vi "New Main Log Loop.vi"() -> ()   [LabVIEW 2015]
uses:
  Old code/packet types.ctl
  frc-software-2016/Robot/Main/Robot Global Data.vi
  <vilib>/Rock Robotics/WPI/Solenoid/Deprecated/WPI_SolenoidGetBool.vi
  frc-software-2016/Sprocket/lib/Sprocket.lvlib
  frc-software-2016/Sprocket/src/Refname/Actuators.ctl
panel:
  out "error out":errorcluster
  out "result string":string
  in  "error in (no error)":errorcluster
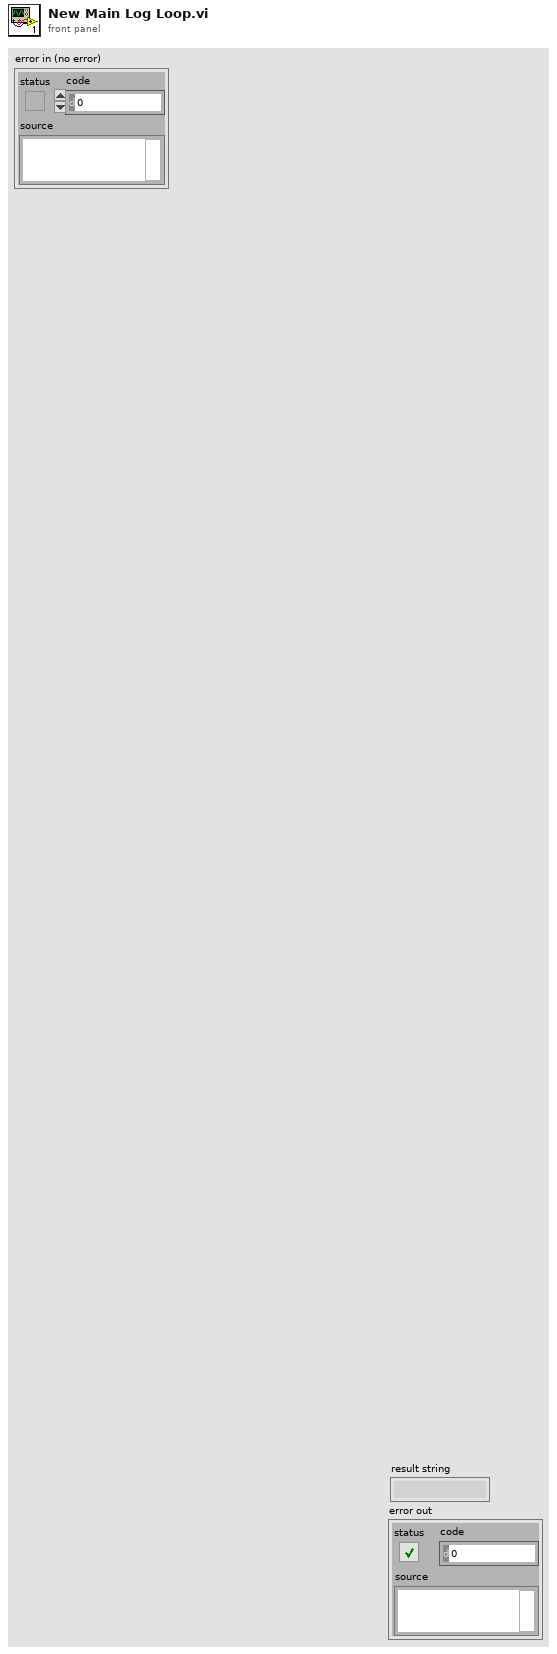
[diagram p1: front panel]
types:
  T1 = typedef "Sprocket.lvlib/Actuators.ctl" = enum16{"Drive Motors L.Top", "Drive Motors R.Top", "Drive Motors L.Bot", "Drive Motors R.Bot", "Collector Motor", "Collector Solenoid", "Compressor", "SonicShifter"}
  T2 = typedef "packet types.ctl" = enum16{"Log line", "Open File", "Send Header", "Set Time", "Send to LCD"}
  T3 = typedef "WPI_SerialPortRef.ctl" = cluster{"DevStatus":errorcluster, "Serial Port Name":refnum<visa-resource-name>}
  T4 = typedef "WPI_MotorControlDeviceRef.ctl" = cluster{"DeviceStatus":errorcluster, "Type":T5, "PWM":cluster{"PWM Channel":T6, "DeadBand":T7}, "CAN":cluster{"Device Number":u8, "Control Mode":T8, "Semaphore":T9, "Max Vout":dbl, "TalonSRX Control Mode":T10}, "Invert":bool}
  T5 = typedef "WPI_MotorControlType.ctl" = enum16{"PWM", "CAN", "CANTalonSRX"}
  T6 = typedef "FPGA_DIOPWMChannel.ctl" = enum8{"PWM 0", "PWM 1", "PWM 2", "PWM 3", "PWM 4", "PWM 5", "PWM 6", "PWM 7", "PWM 8", "PWM 9", "PWM MXP 0", "PWM MXP 1", "PWM MXP 2", "PWM MXP 3", "PWM MXP 4", "PWM MXP 5", "PWM MXP 6", "PWM MXP 7", "PWM MXP 8", "PWM MXP 9", "Invalid"}
  T7 = typedef "WPI_PWMDeadband.ctl" = cluster{"Name":string, "maxPositivePwm":i32, "minPositivePwm":i32, "centerPwm":i32, "maxNegativePwm":i32, "minNegativePwm":i32, "angularRange":u16}
  T8 = typedef "WPI_CANJaguar_ControlMode.ctl" = enum8{"Percent VBus", "Current", "Speed", "Position", "Voltage"}
  T9 = typedef "Semaphore RefNum" = refnum<k1>
  T10 = typedef "WPI_CANTalonSRX_APIControlMode.ctl" = enum8{"Percent VBus", "Speed", "Position", "Slave", "Unchanged / Invalid", "Voltage Compensation", "Current", "Motion Profile"}
  T11 = typedef "WPI_CompressorDevRef.ctl" = cluster{"DevStatus":errorcluster, "Pneumatics Control Module":u8}
  T12 = typedef "WPI_SolenoidDevRef.ctl" = cluster{"DevStatus":errorcluster, "Pneumatics Control Module":u8, "Forward Solenoid Channel":T13, "Reverse Solenoid Channel":T13}
  T13 = typedef "WPI_SolenoidChannel.ctl" = enum8{"Solenoid 0", "Solenoid 1", "Solenoid 2", "Solenoid 3", "Solenoid 4", "Solenoid 5", "Solenoid 6", "Solenoid 7", "Invalid"}
  T14 = typedef "WPI_DriverStationRobotMode2.ctl" = enum16{"Autonomous Disabled", "Autonomous Enabled", "Teleop Disabled", "Teleop Enabled", "Disconnected", "Finish", "Test Disabled", "Test Enabled", "Emergency Stopped"}
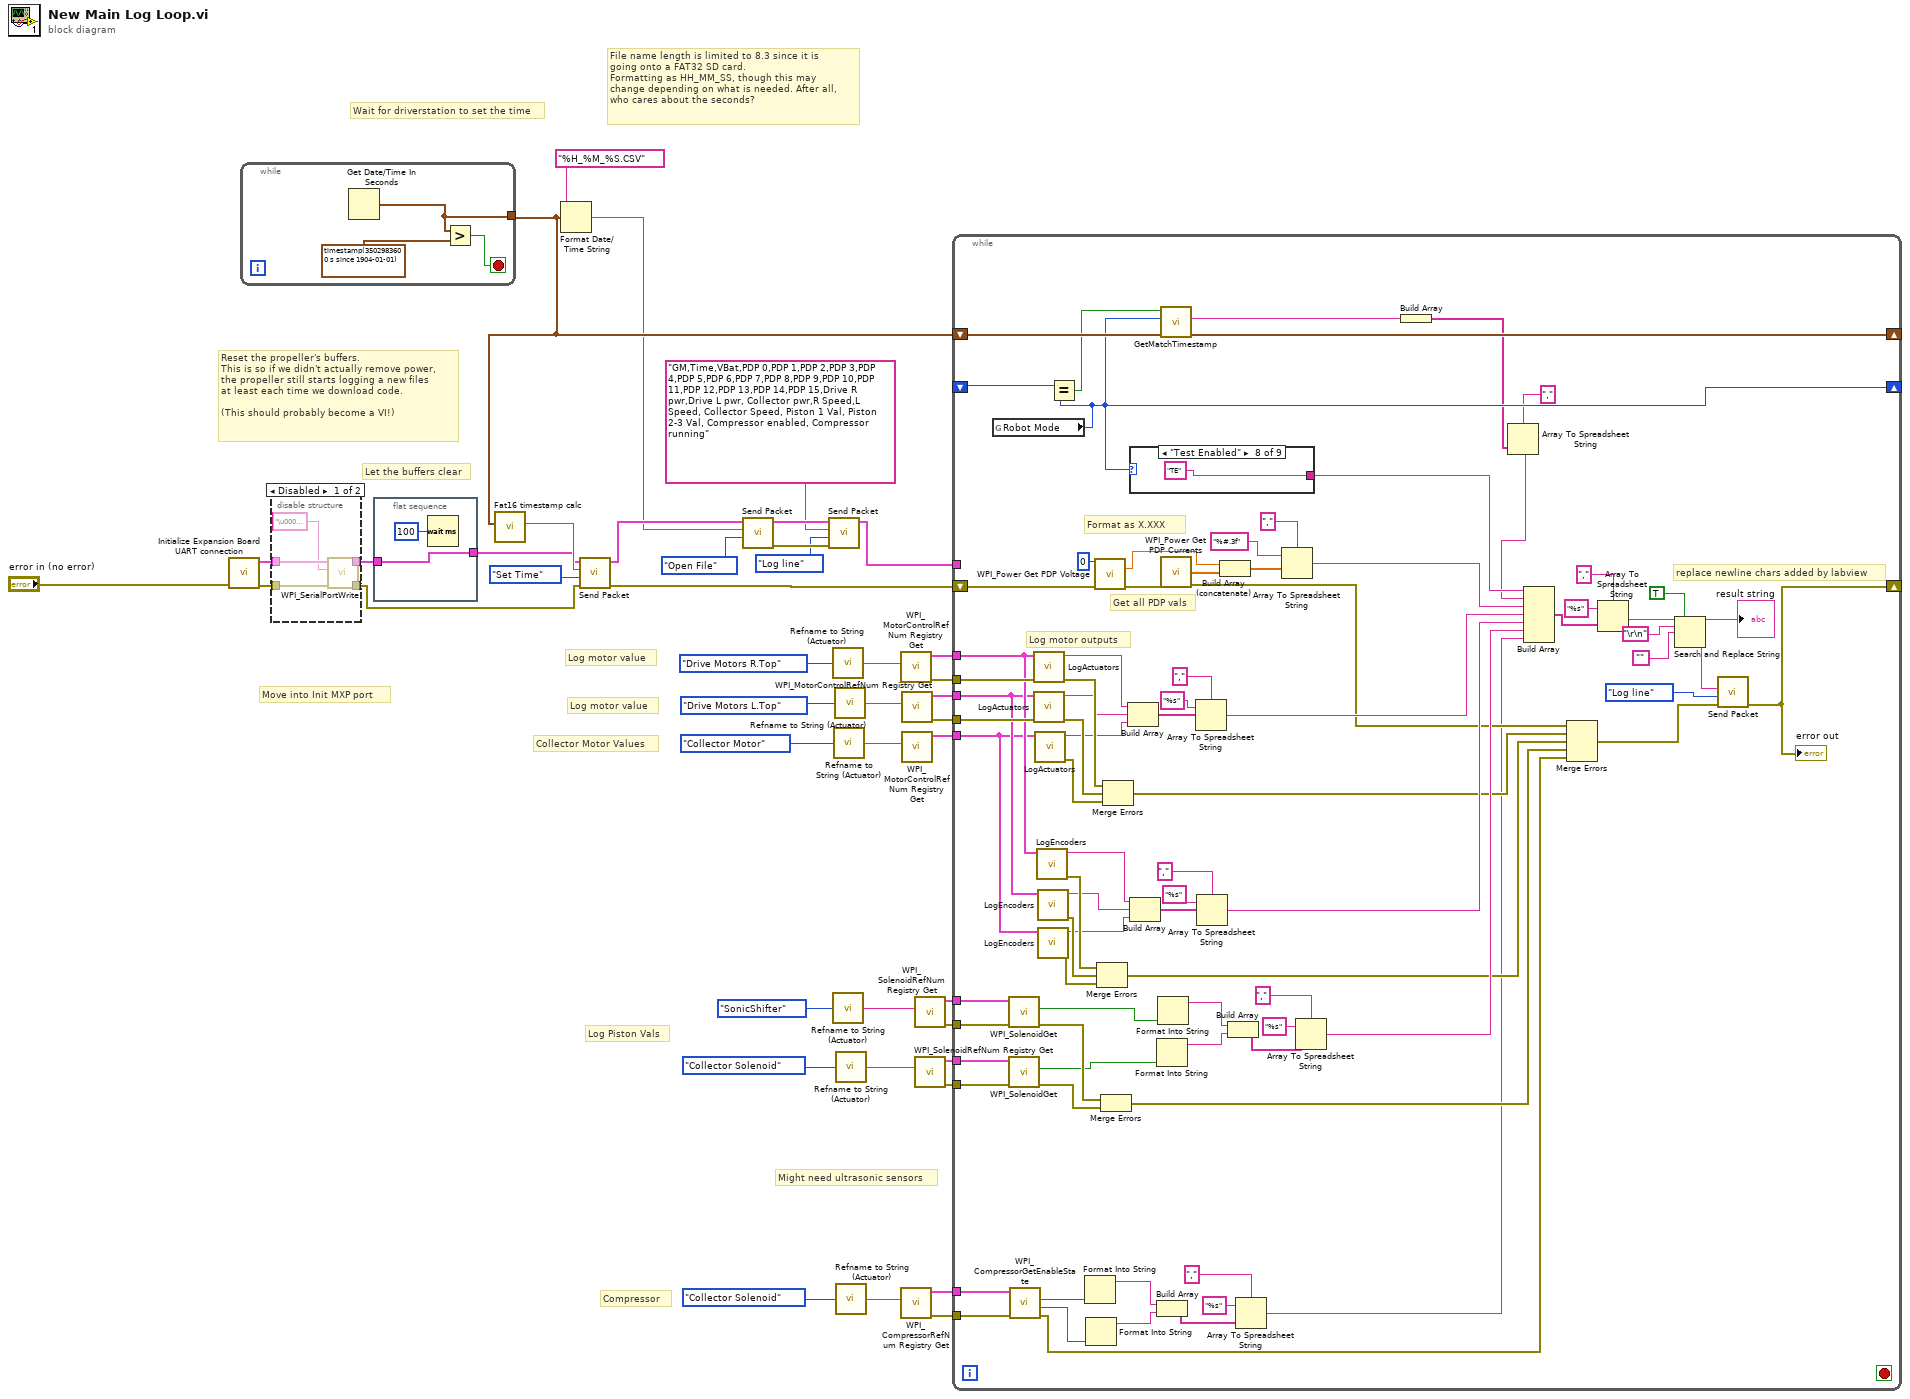
[diagram p0: block diagram]
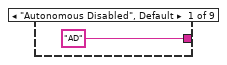
[diagram p2: hidden frame]
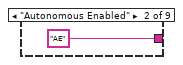
[diagram p3: hidden frame]
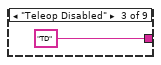
[diagram p4: hidden frame]
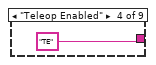
[diagram p5: hidden frame]
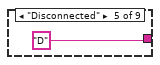
[diagram p6: hidden frame]
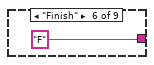
[diagram p7: hidden frame]
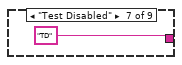
[diagram p8: hidden frame]
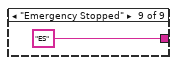
[diagram p9: hidden frame]
diagram:
  # "Might need ultrasonic sensors"
  # "Collector Motor Values"
  # "Compressor"
  # "Log motor value"
  # "Log motor value"
  # "Log Piston Vals"
  # "Move into Init MXP port"
  # "Let the buffers clear"
  # "Reset the propeller's buffers.\nThis is so if we didn't actually remove power,\nthe propeller still starts logging a new files \nat least each time we download code.\n\n(This should probably become a VI!)"
  # "File name length is limited to 8.3 since it is \ngoing onto a FAT32 SD card. \nFormatting as HH_MM_SS, though this may\nchange depending on what is needed. After all,\nwho cares about the seconds?"
  # "Wait for driverstation to set the time"
  n1 = call "Initialize Expansion Board UART connection.vi"("error in (no error)"="error in (no error)") -> ("error out"=w39:errorcluster, "SerialPortRef"=w38:T3)  [unwired: 9 in]
  n2 = while {
    tunnel: [w43] -> w33
    stop <- w44 stop-if-true
    n3 = Get Date/Time In Seconds() -> (seconds since 1Jan1904=w43:timestamp)
    n4 = Greater?(x=w43, y=timestamp(3502983600 s since 1904-01-01)) -> (0:w44:bool)
  }
  n5 = disable-structure shown="Disabled" {
    disable-tunnel: w39 -> [w50 w51]
    disable-tunnel: w38 -> [w49 w52]
    disable-tunnel: [w47 w52] -> w36
    disable-tunnel: [w46 w51] -> w35
    frame Disabled {
      n6 = call <vilib>:"WPI_SerialPortWrite.vi"("error in (no error)"=w50, "Buffer"="\u0004\u0004", "SerialPortRef"=w49) -> ("error out"=w46:errorcluster, "SerialPortRef"=w47:T3)  [unwired: 6 in, 1 out]
    }
    frame Enabled {
    }
  }
  n7 = flat-sequence {
    tunnel: [w54] -> w37
    tunnel: w36 -> [w54]
    frame #0 {
      n8 = Wait (ms)(milliseconds to wait=u32 100) -> ()  [unwired: 1 out]
    }
  }
  n9 = call "Fat16 timestamp calc.vi"("time stamp"=w33) -> ("timestamp as string"=w41:string)  [unwired: 10 in]
  n10 = Format Date/Time String(time format string (%c)="%H_%M_%S.CSV", seconds (now)=w33) -> (date/time string=w26:string)  [unwired: 1 in]
  n11 = call "Send Packet.vi"("error in (no error)"=w35, 7:packet_types."Set Time", "Log string"=w41, "SerialPortRef"=w37) -> ("error out"=w24:errorcluster, "SerialPortRef out"=w27:T3)  [unwired: 4 in]
  n12 = call "Send Packet.vi"(7:packet_types."Open File", "Log string"=w26, "SerialPortRef"=w27) -> ("error out"=w31:errorcluster, "SerialPortRef out"=w32:T3)  [unwired: 5 in]
  n13 = call "Send Packet.vi"("error in (no error)"=w31, 7:packet_types."Log line", "Log string"="GM,Time,VBat,PDP 0,PDP 1,PDP 2,PDP 3,PDP 4,PDP 5,PDP 6,PDP 7,PDP 8,PDP 9,PDP 10,PDP 11,PDP 12,PDP 13,PDP 14,PDP 15,Drive R pwr,Drive L pwr, Collector pwr,R Speed,L Speed, Collector Speed, Piston 1 Val, Piston 2-3 Val, Compressor enabled, Compressor running", "SerialPortRef"=w32) -> ("SerialPortRef out"=w28:T3)  [unwired: 4 in, 1 out]
  n14 = call "Refname to String (Actuator).vi"("Actuator Refname"=Actuators."Drive Motors R.Top") -> ("Refnum Name"=w21:string)
  n15 = call "Refname to String (Actuator).vi"("Actuator Refname"=Actuators."SonicShifter") -> ("Refnum Name"=w11:string)
  n16 = call "Refname to String (Actuator).vi"("Actuator Refname"=Actuators."Collector Motor") -> ("Refnum Name"=w14:string)
  n17 = call "Refname to String (Actuator).vi"("Actuator Refname"=Actuators."Drive Motors L.Top") -> ("Refnum Name"=w19:string)
  n18 = call "Refname to String (Actuator).vi"("Actuator Refname"=Actuators."Collector Solenoid") -> ("Refnum Name"=w7:string)
  n19 = call "Refname to String (Actuator).vi"("Actuator Refname"=Actuators."Collector Solenoid") -> ("Refnum Name"=w2:string)
  n20 = call <vilib>:"WPI_MotorControlRefNum Registry Get.vi"("refnum name"=w21) -> ("error out"=w17:errorcluster, "MotorControlDevRef"=w22:T4)  [unwired: 9 in]
  n21 = call <vilib>:"WPI_CompressorRefNum Registry Get.vi"("refnum name"=w2) -> ("error out"=w1:errorcluster, "CompressorDevRef"=w3:T11)  [unwired: 9 in]
  n22 = call <vilib>:"WPI_MotorControlRefNum Registry Get.vi"("refnum name"=w19) -> ("error out"=w16:errorcluster, "MotorControlDevRef"=w18:T4)  [unwired: 9 in]
  n23 = call <vilib>:"WPI_MotorControlRefNum Registry Get.vi"("refnum name"=w14) -> ("MotorControlDevRef"=w13:T4)  [unwired: 9 in, 1 out]
  n24 = call <vilib>:"WPI_SolenoidRefNum Registry Get.vi"("refnum name"=w11) -> ("error out"=w9:errorcluster, "SolenoidDevRef"=w10:T12)  [unwired: 9 in]
  n25 = call <vilib>:"WPI_SolenoidRefNum Registry Get.vi"("refnum name"=w7) -> ("error out"=w5:errorcluster, "SolenoidDevRef"=w8:T12)  [unwired: 9 in]
  n26 = while {
    shift-right: [w135] -> _
    shift-left: w33 -> [w134]
    shift-right: [w131] -> _
    shift-left: _ -> [w133]
    tunnel: w28 -> [_]
    tunnel: w18 -> [w62]
    tunnel: w8 -> [w104]
    shift-right: [w81] -> _
    shift-left: w24 -> [w80]
    tunnel: w3 -> [w79]
    tunnel: w17 -> [w65]
    tunnel: w22 -> [w63]
    tunnel: w16 -> [w64]
    tunnel: w13 -> [w61]
    tunnel: w10 -> [w60]
    tunnel: w9 -> [w59]
    tunnel: w5 -> [w58]
    tunnel: w1 -> [w55]
    stop <- _ stop-if-true
    # "Get all PDP vals"
    # "replace newline chars added by labview"
    # "Log motor outputs"
    # "Format as X.XXX"
    n27 = global read "Robot Global Data.vi" "Robot Mode"() -> (w131:T14)
    n28 = call-poly <vilib>:"WPI_SolenoidGet.vi"("error in (no error)"=w59, "SolenoidDevRef"=w60) -> ("error out"=w102:errorcluster, "Value"=w101:bool)  [unwired: 7 in, 1 out]
    n29 = call-poly <vilib>:"WPI_SolenoidGet.vi"("error in (no error)"=w58, "SolenoidDevRef"=w104) -> ("error out"=w103:errorcluster, "Value"=w100:bool)  [unwired: 7 in, 1 out]
    n30 = call <vilib>:"WPI_CompressorGetEnableState.vi"("error in (no error)"=w55, "CompressorDevRef"=w79) -> ("error out"=w57:errorcluster, "Compressor Running"=w73:bool, "Enabled"=w74:bool)  [unwired: 6 in, 1 out]
    n31 = call "LogActuators.vi"("error in (no error) 2"=w65, "MotorControlDevRef"=w63) -> ("error out"=w112:errorcluster, "resulting string"=w109:string)  [unwired: 8 in]
    n32 = call "LogActuators.vi"("error in (no error) 2"=w64, "MotorControlDevRef"=w62) -> ("error out"=w113:errorcluster, "resulting string"=w108:string)  [unwired: 8 in]
    n33 = call "LogActuators.vi"("MotorControlDevRef"=w61) -> ("error out"=w114:errorcluster, "resulting string"=w107:string)  [unwired: 9 in]
    n34 = call "LogEncoders.vi"("CAN Talon SRX Ref"=w63) -> ("error out"=w138:errorcluster, "concatenated string"=w127:string)  [unwired: 9 in]
    n35 = call "LogEncoders.vi"("CAN Talon SRX Ref"=w62) -> ("error out"=w137:errorcluster, "concatenated string"=w126:string)  [unwired: 9 in]
    n36 = call "LogEncoders.vi"("CAN Talon SRX Ref"=w61) -> ("error out"=w136:errorcluster, "concatenated string"=w125:string)  [unwired: 9 in]
    n37 = Equal?(x=w133, y=w131) -> (x = y?=w132:bool)
    n38 = Format Into String(w74) -> (resulting string=w77:string)  [unwired: 3 in, 1 out]
    n39 = Format Into String(w73) -> (resulting string=w76:string)  [unwired: 3 in, 1 out]
    n40 = call <vilib>:"WPI_Power Get PDP Voltage.vi"("Power Distribution Panel (0)"=u8 0, "error in"=w80) -> ("voltage (V)"=w121:dbl, "error out"=w118:errorcluster)  [unwired: 12 in]
    n41 = Merge Errors(w138, w137, w136) -> (w84:errorcluster)
    n42 = Merge Errors(w102, w103) -> (w83:errorcluster)
    n43 = Merge Errors(w112, w113, w114) -> (w85:errorcluster)
    n44 = Build Array(w109, w108, w107) -> (w111:string[])
    n45 = case shown="\"Test Enabled\"" w131 {
      tunnel: ["AD" "AE" "TD" "TE" "D" "F" "TD" "TE" "ES"] -> w130
      frame "Autonomous Disabled", Default {
      }
      frame "Autonomous Enabled" {
      }
      frame "Teleop Disabled" {
      }
      frame "Teleop Enabled" {
      }
      frame "Disconnected" {
      }
      frame "Finish" {
      }
      frame "Test Disabled" {
      }
      frame "Test Enabled" {
      }
      frame "Emergency Stopped" {
      }
    }
    n46 = Build Array(w127, w126, w125) -> (w129:string[])
    n47 = Format Into String(w100) -> (resulting string=w97:string)  [unwired: 3 in, 1 out]
    n48 = Build Array(w77, w76) -> (w78:string[])
    n49 = Format Into String(w101) -> (resulting string=w98:string)  [unwired: 3 in, 1 out]
    n50 = call "GetMatchTimestamp.vi"("seconds since 1Jan1904"=w134, "Robot Mode"=w131, "Boolean"=w132) -> ("seconds since 1Jan1904 2"=w135:timestamp, "Match Timestamp"=w67:string)  [unwired: 7 in]
    n51 = call <vilib>:"WPI_Power Get PDP Currents.vi"("error in"=w118) -> ("all currents (A)"=w119:dbl[], "error out"=w86:errorcluster)  [unwired: 12 in, 1 out]
    n52 = Array To Spreadsheet String(delimiter (Tab)=",", array=w111, 3:"%s" ("format string")) -> (spreadsheet string=w105:string)
    n53 = Array To Spreadsheet String(delimiter (Tab)=",", array=w129, 3:"%s" ("format string")) -> (spreadsheet string=w106:string)
    n54 = Build Array (concatenate)(w121, w119) -> (w120:dbl[])
    n55 = Build Array(w98, w97) -> (w99:string[])
    n56 = Array To Spreadsheet String(delimiter (Tab)=",", array=w78, 3:"%s" ("format string")) -> (spreadsheet string=w56:string)
    n57 = Array To Spreadsheet String(delimiter (Tab)=",", array=w120, 3:"%#.3f" ("format string")) -> (spreadsheet string=w117:string)
    n58 = Array To Spreadsheet String(delimiter (Tab)=",", array=w99, 3:"%s" ("format string")) -> (spreadsheet string=w95:string)
    n59 = Build Array(w67) -> (w66:string[])
    n60 = Array To Spreadsheet String(delimiter (Tab)=",", array=w66) -> (spreadsheet string=w116:string)  [unwired: 1 in]
    n61 = Build Array(w130, w116, w117, w105, w106, w95, w56) -> (w89:string[])
    n62 = Merge Errors(w86, w85, w84, w83, w57) -> (w82:errorcluster)
    n63 = Array To Spreadsheet String(delimiter (Tab)=",", array=w89, 3:"%s" ("format string")) -> (spreadsheet string=w90:string)
    n64 = Search and Replace String(replace all?=TRUE ("replace all? (F)"), input string=w90, search string="\r\n", replace string="") -> (result string=w88:string)  [unwired: 4 in, 3 out]
    "result string" <- w88
    n65 = call "Send Packet.vi"("error in (no error)"=w82, 7:packet_types."Log line", "Log string"=w88) -> ("error out"=w81:errorcluster)  [unwired: 5 in, 1 out]
    "error out" <- w81
  }
